vi "niDTS BT Tx Test UTIL EDR DEVM Parameters to BT ModAcc Parameters.vi"(7 "ModAcc Measurement Paramaters in":T1={"DEVM Enable"=FALSE, "Averages"=1, "Averaging Mode"=enum."RMS", "Measurement Duration (bytes)"=-1, "Measurement Offset (bytes)"=0}) -> (8 "ModAcc Measurement Paramaters out":T2={"ModAcc Enable"=FALSE, "CFO Enable"=FALSE, "Character Select"=enum."DF1", "Averages"=1, "Averaging Mode"=enum."RMS", "Measurement Duration"=-1, "Measurement Offset"=0})   [LabVIEW 2015, in "niDTS BT.lvlib"]
uses:
  niDTS BT.lvlib
  Includes/niDTS BT INC EDR ModAcc Measurement Parameters.ctl
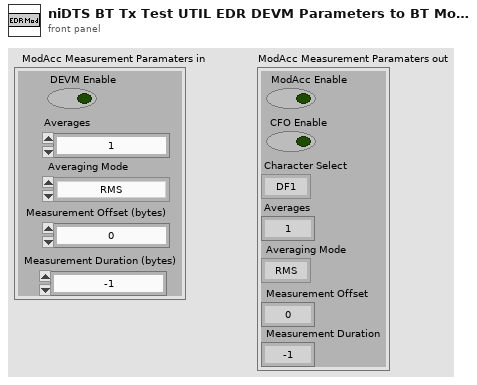
[diagram p1: front panel]
types:
  T1 = typedef "niDTS BT.lvlib/niDTS BT INC EDR ModAcc Measurement Parameters.ctl" = cluster{"DEVM Enable":bool, "Averages":i32, "Averaging Mode":enum16{"RMS", "LOG", "SCALAR", "MAX", "MIN", "VECTOR"}, "Measurement Duration (bytes)":i32, "Measurement Offset (bytes)":i32}
  T2 = cluster{"ModAcc Enable":bool, "CFO Enable":bool, "Character Select":enum16{"DF1", "DF2"}, "Averages":i32, "Averaging Mode":enum16{"RMS", "LOG", "SCALAR", "MAX", "MIN", "VECTOR"}, "Measurement Duration":i32, "Measurement Offset":i32}
  T3 = enum16{"RMS", "LOG", "SCALAR", "MAX", "MIN", "VECTOR"}
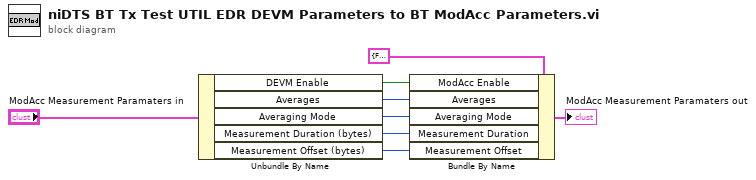
[diagram p0: block diagram]
diagram:
  n1 = Unbundle By Name("ModAcc Measurement Paramaters in") -> ("DEVM Enable"=w3:bool, "Averages"=w4:i32, "Averaging Mode"=w5:T3, "Measurement Duration (bytes)"=w6:i32, "Measurement Offset (bytes)"=w7:i32)
  n2 = Bundle By Name(cluster=T2 {"ModAcc Enable"=FALSE, "CFO Enable"=FALSE, "Character Select"=enum."DF1", "Averages"=0, "Averaging Mode"=enum."RMS", "Measurement Duration"=0, "Measurement Offset"=0} ("ModAcc Measurement Paramaters 2"), "ModAcc Enable"=w3, "Averages"=w4, "Averaging Mode"=w5, "Measurement Duration"=w6, "Measurement Offset"=w7) -> (→"ModAcc Measurement Paramaters out":T2)
